vi "read_Xred.vi"(8 "error in (no error)":errorcluster, 11 "FeatureAgglomeration in":refnum<class "FeatureAgglomeration.lvclass">) -> (0 "error out":errorcluster, 2 "Xred":dbl[][](array[numeric]), 3 "FeatureAgglomeration out":refnum<class "FeatureAgglomeration.lvclass">)   [LabVIEW 2020, in "FeatureAgglomeration.lvclass"]
uses:
  FeatureAgglomeration.lvclass
  FeatureAgglomeration.lvclass/FeatureAgglomeration.ctl
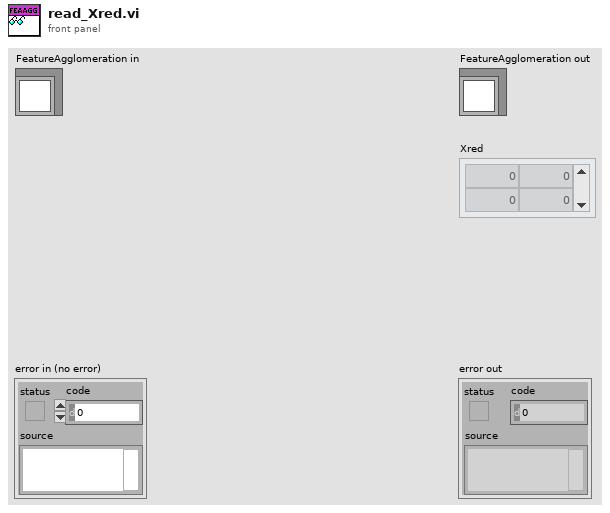
[diagram p1: front panel]
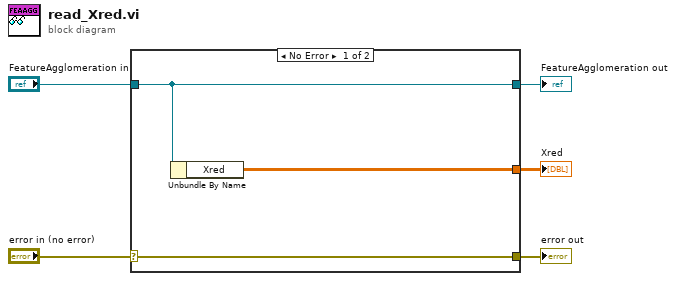
[diagram p0: block diagram]
diagram:
  n1 = case shown="No Error" "error in (no error)" {
    selector: "error in (no error)" -> [w8 w9]
    tunnel: [w8 w9] -> w4
    tunnel: [w7 w10] -> w2
    tunnel: "FeatureAgglomeration in" -> [w7 w10]
    tunnel: [w6 _] -> w1
    frame No Error {
      n2 = Unbundle By Name(w7) -> ("Xred"=w6:dbl[][])
    }
    frame Error {
    }
  }
  "error out" <- w4
  "FeatureAgglomeration out" <- w2
  "Xred" <- w1
